vi "LED.vi"(6 "Numbers":dbl[](array[numeric])=[2.0, 4.0, 100.0, 30.0, 2.0, 6.0], 8 "colors":u32[](array[colorbox])=[16712704, 1507583, 65302], 9 "Control_State":T1, 10 "Length":dbl, 11 "Iteration_Num":dbl) -> (3 "Output_Array":u32[](array[numeric]))   [LabVIEW 2020]
uses:
  <vilib>/numeric/Random Number (Range) U64.vi
  af1e4812-ce9e-4321-a641-5b8f74c4ca52.vi
  0c29d166-b99e-4576-9ee3-0d9caf6f3888.vi
  LED_Control_States.ctl
panel:
  in  "Flames":u32[](array[colorbox])=[16711680, 16718848, 16727296, 16733696, 16743168, 16750592, 15706624, 16758784, 16768322, 16776704, 0, 0, 0]
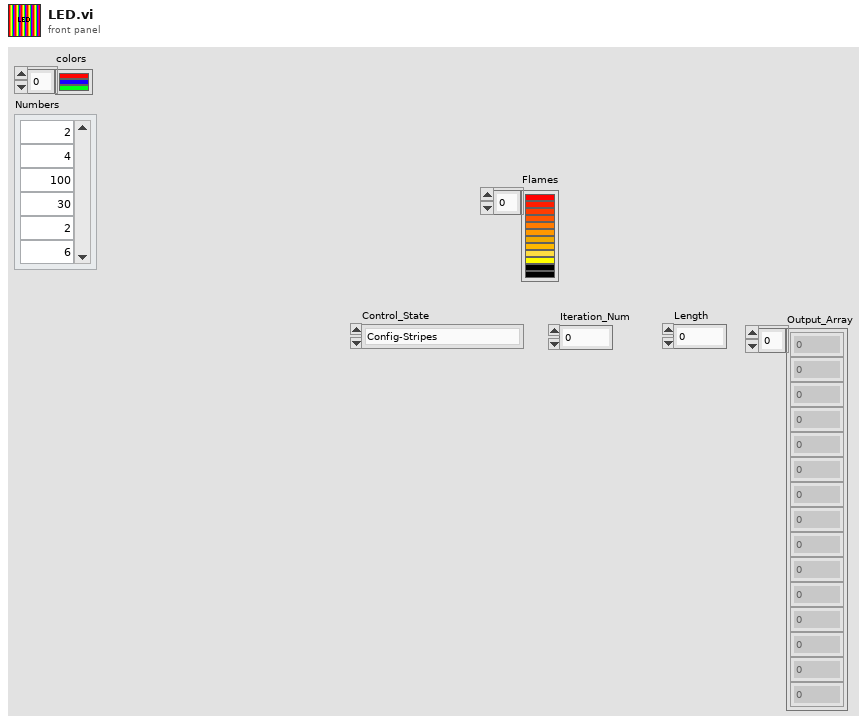
[diagram p1: front panel]
types:
  T1 = typedef "LED_Control_States.ctl" = enum16{"Config-Stripes", "swapperlines", "Rand", "Solid", "Flash-S", "Gradyent", "Move-Stripes", "Org-Rand", "Move-Point-Tail", "Flames", "Fade", "Alt-Colors"}
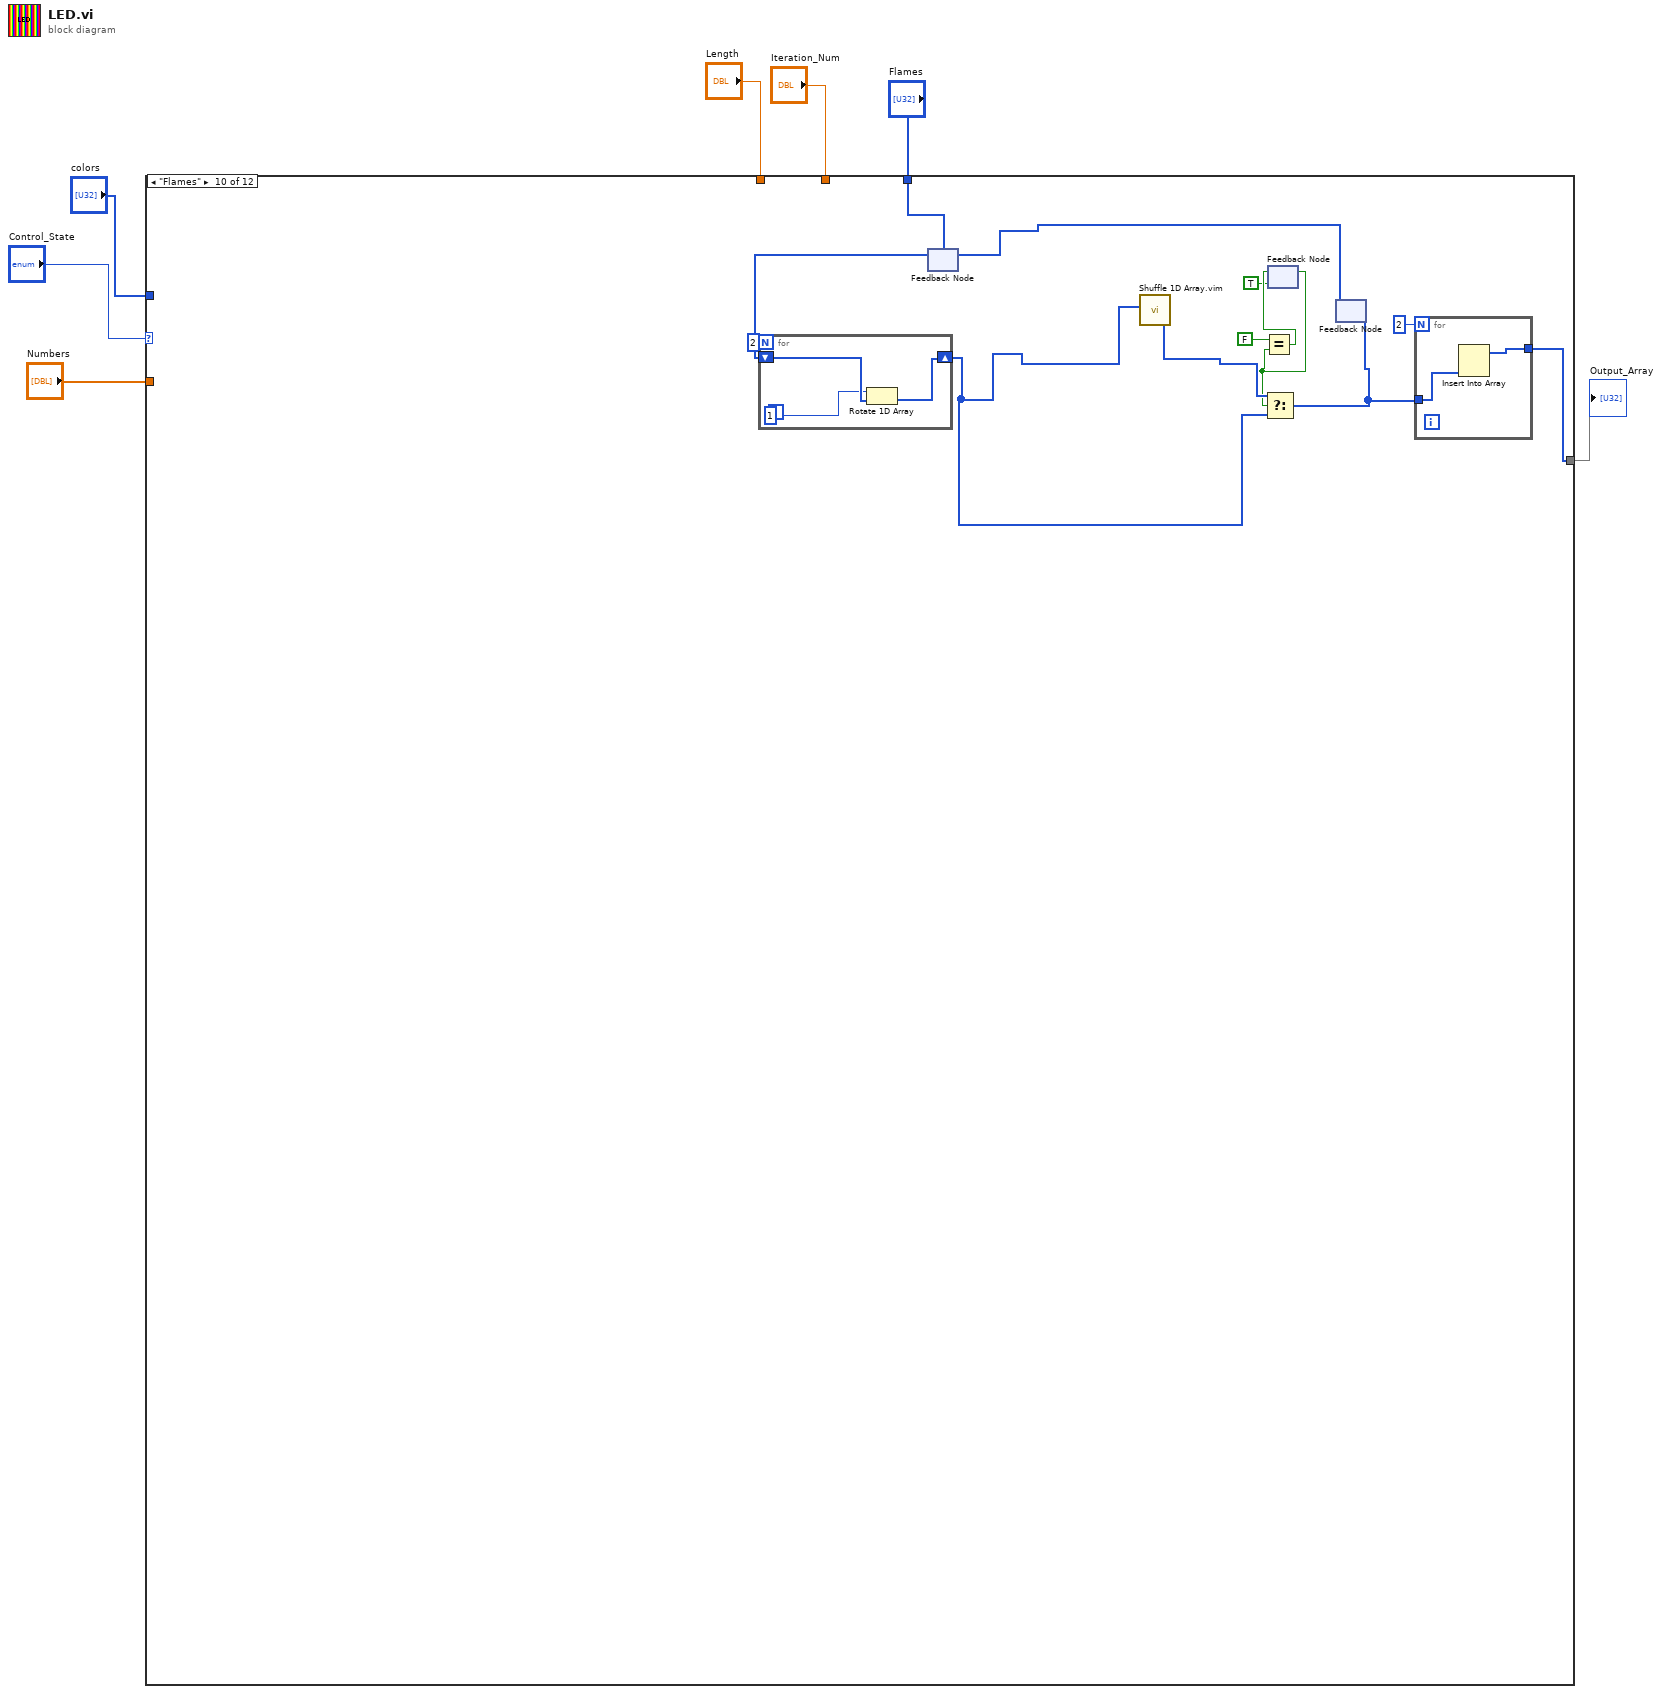
[diagram p0: block diagram]
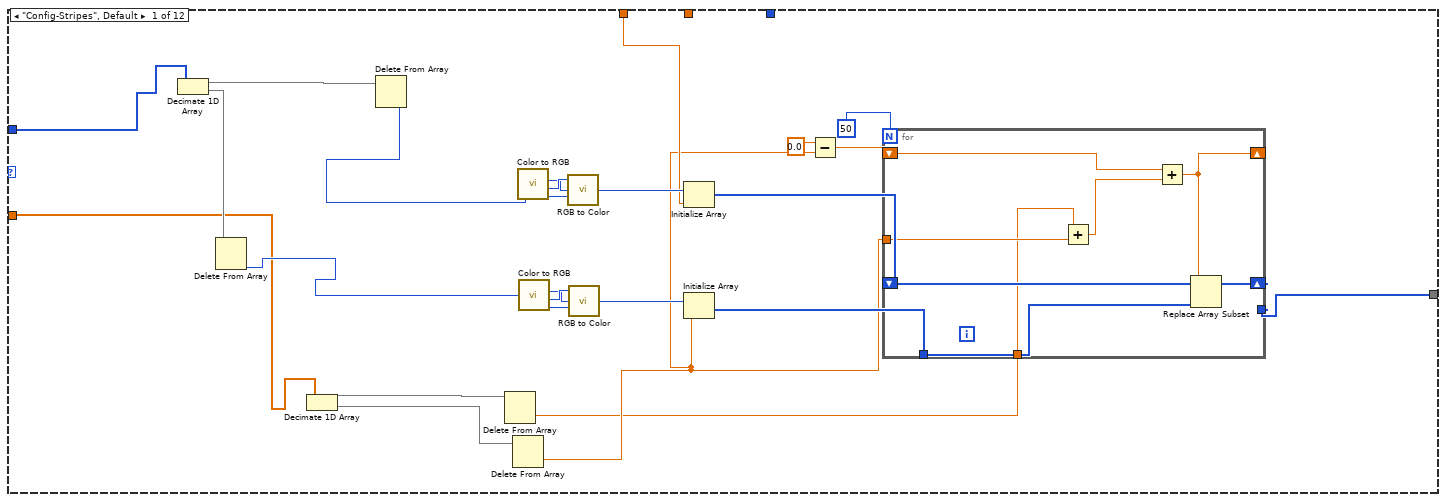
[diagram p2: hidden frame]
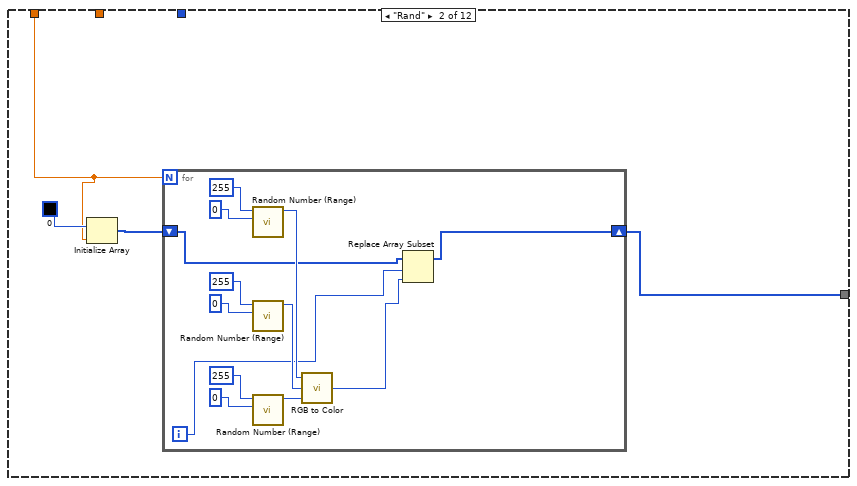
[diagram p3: hidden frame]
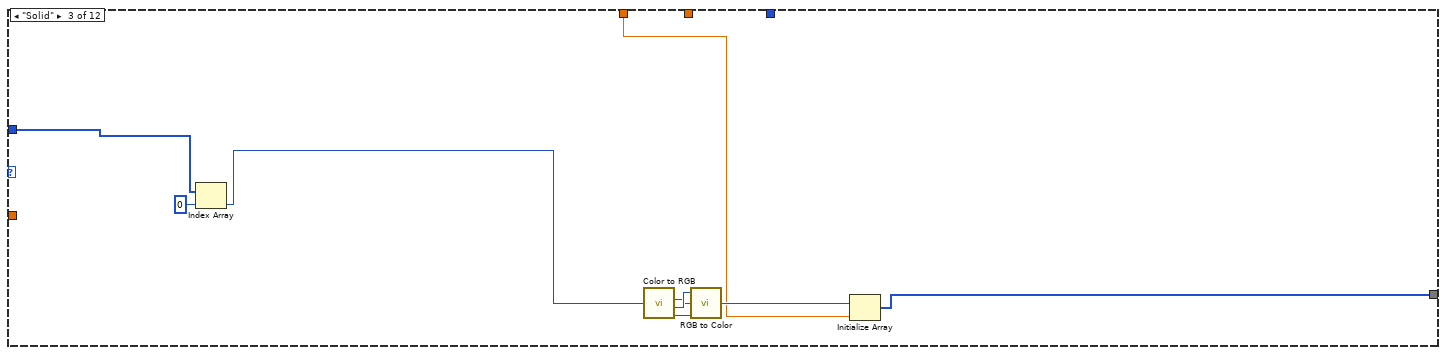
[diagram p4: hidden frame]
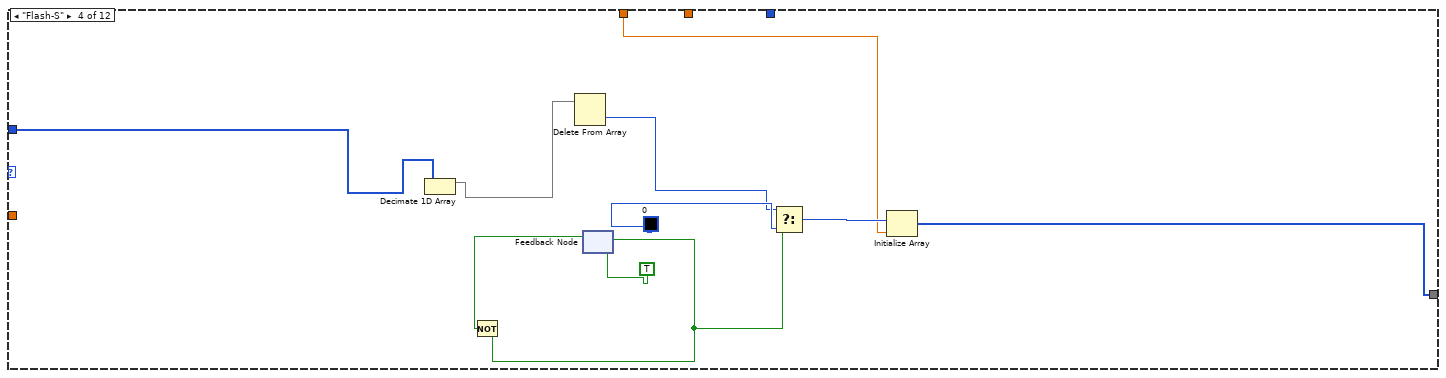
[diagram p5: hidden frame]
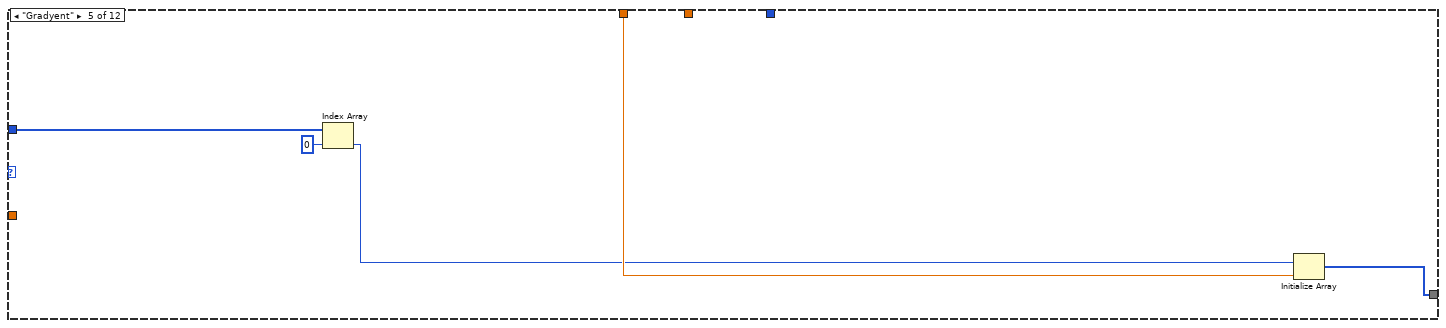
[diagram p6: hidden frame]
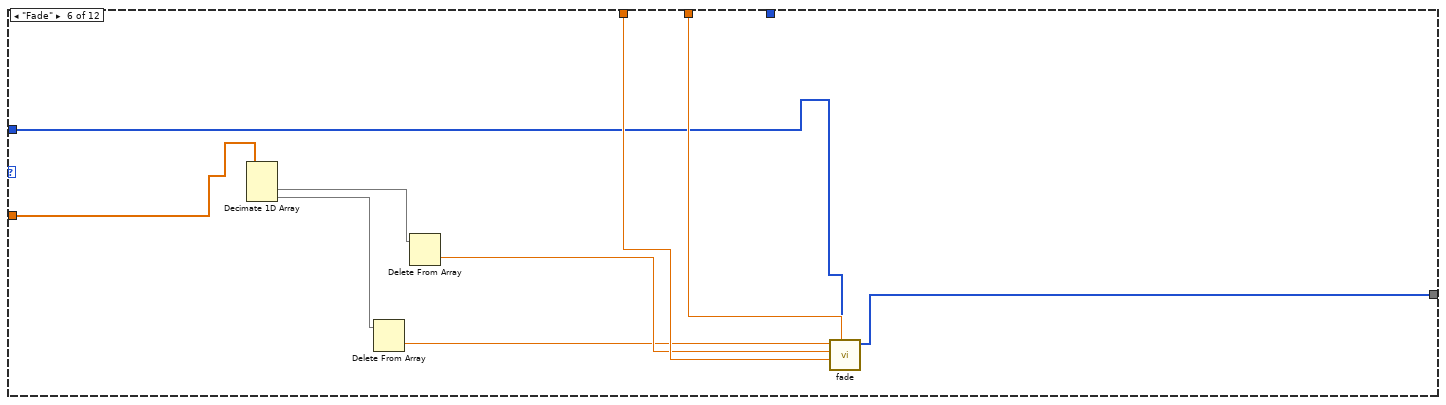
[diagram p7: hidden frame]
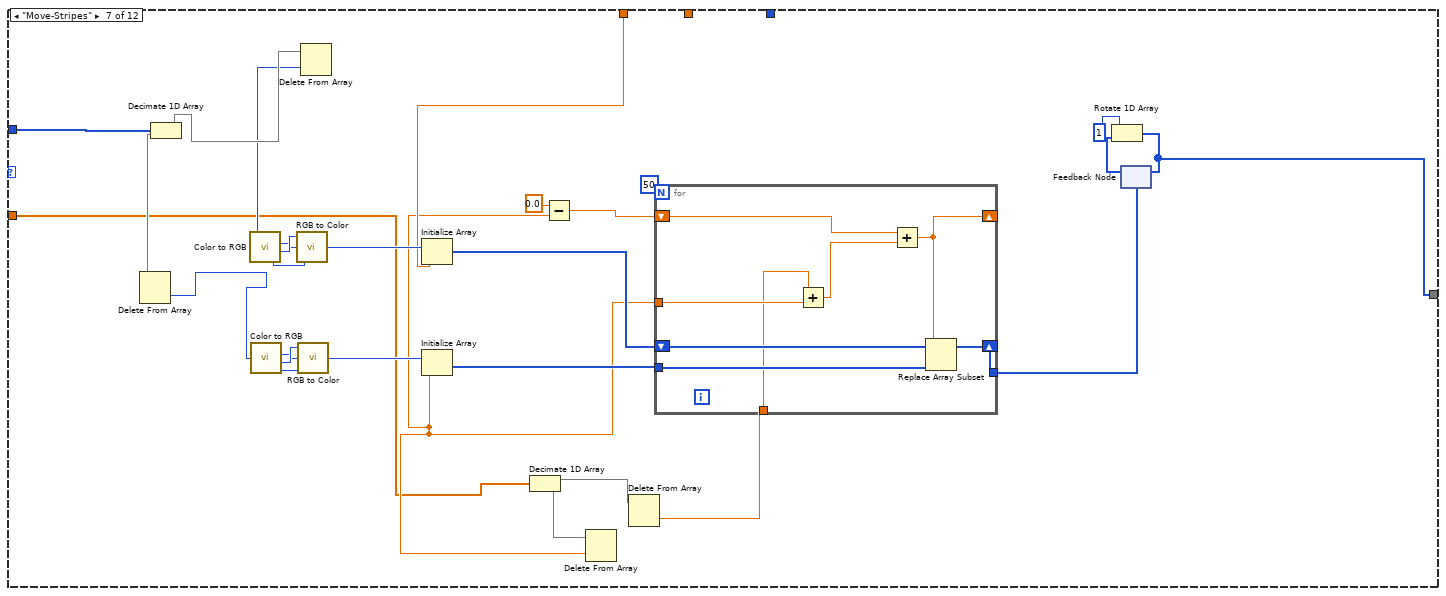
[diagram p8: hidden frame]
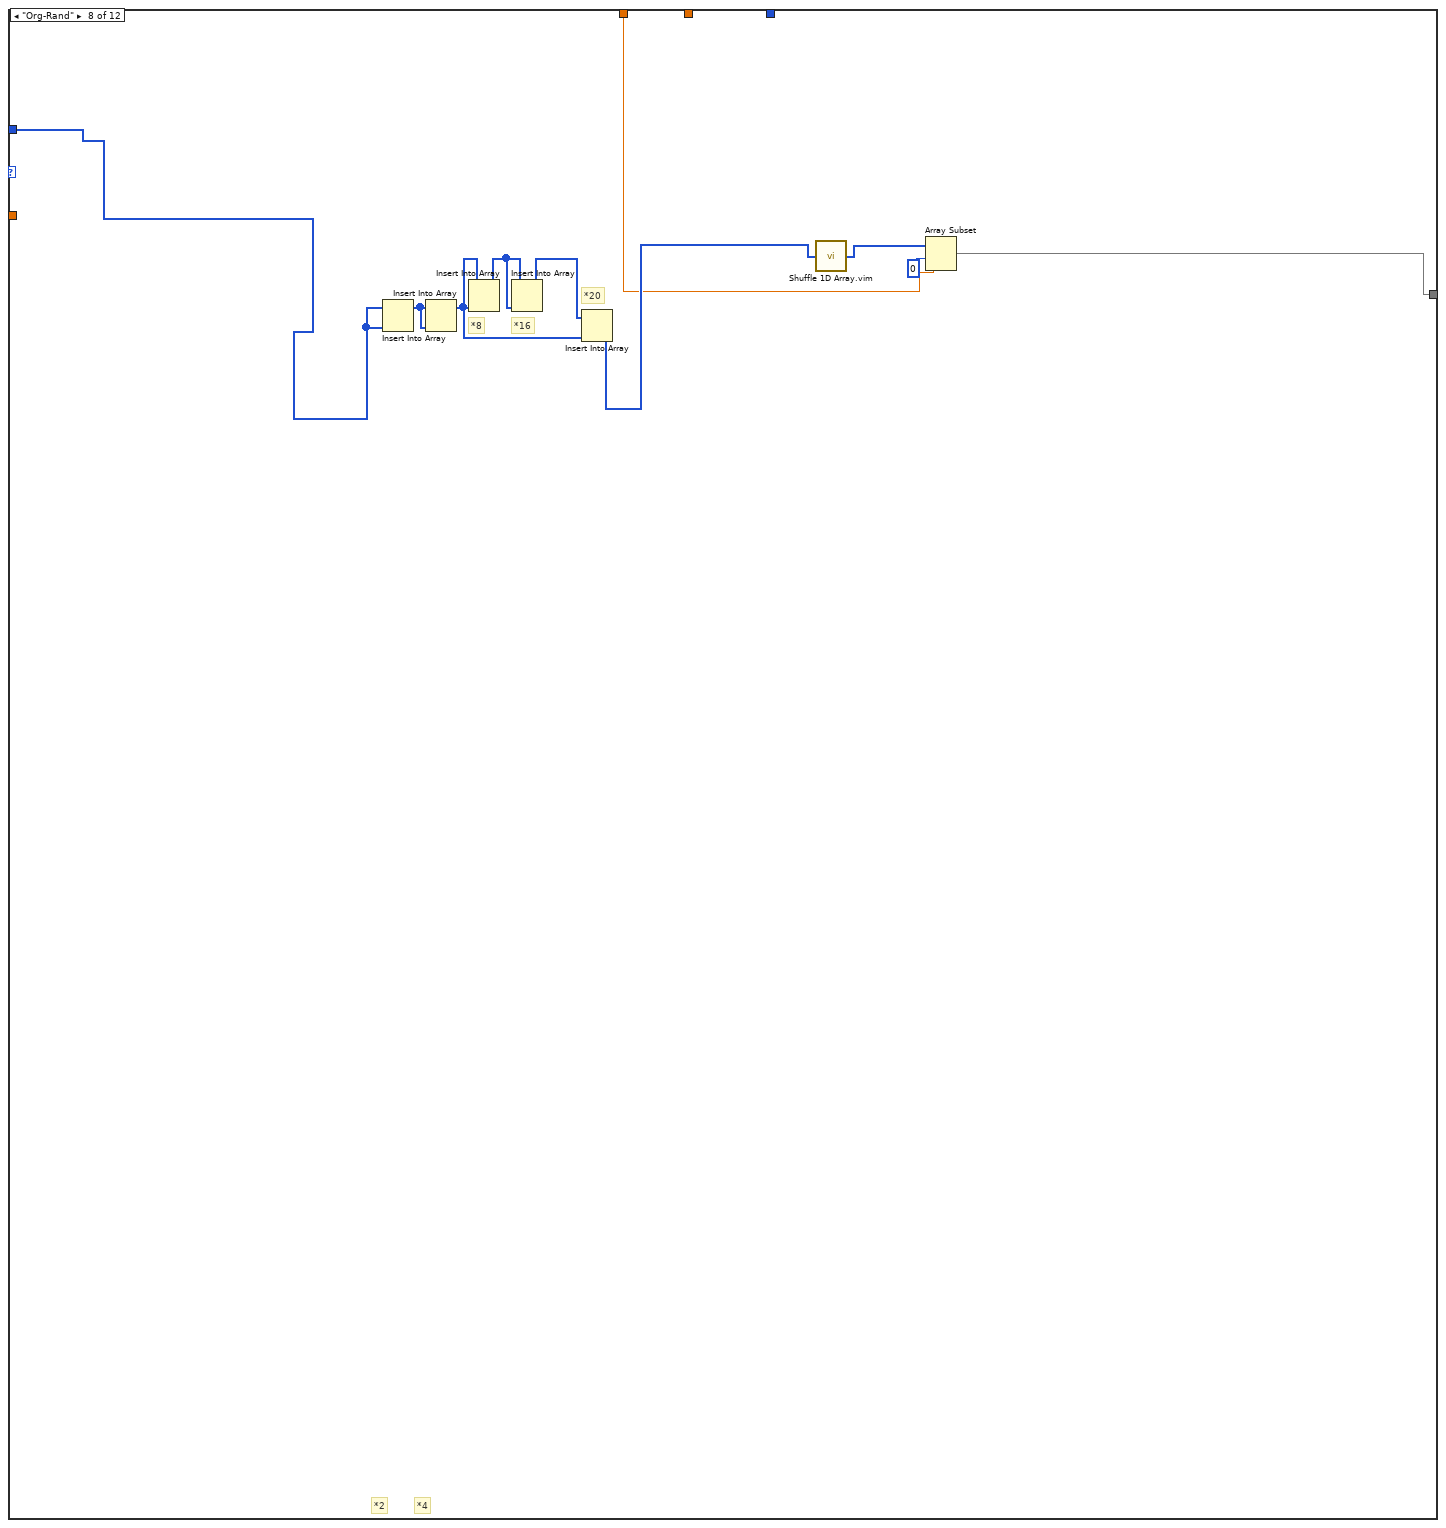
[diagram p9: hidden frame]
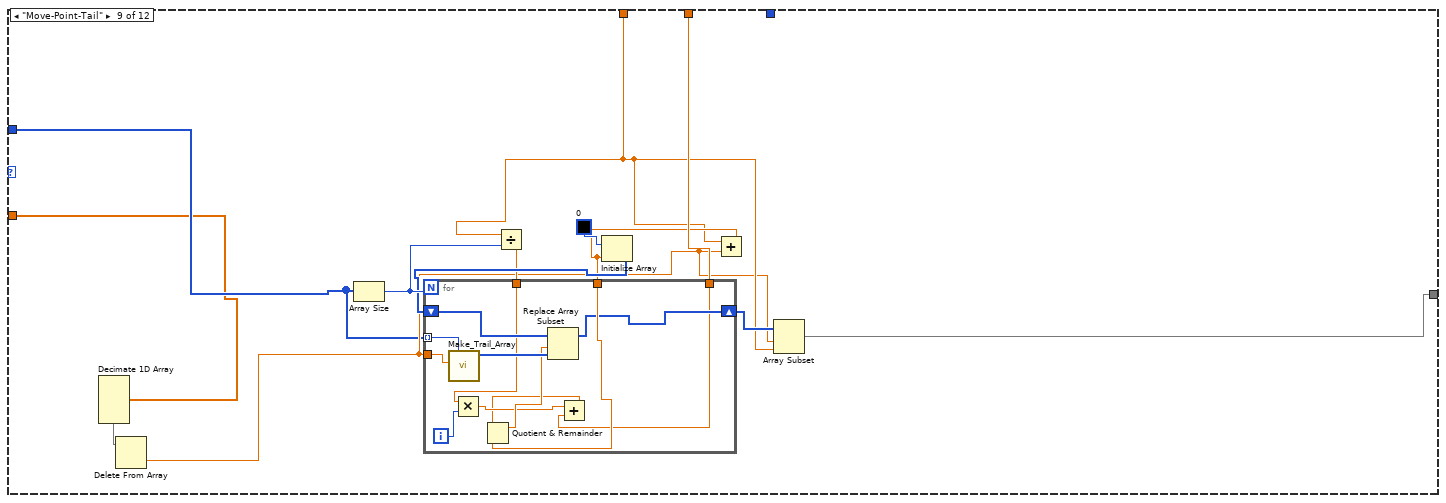
[diagram p10: hidden frame]
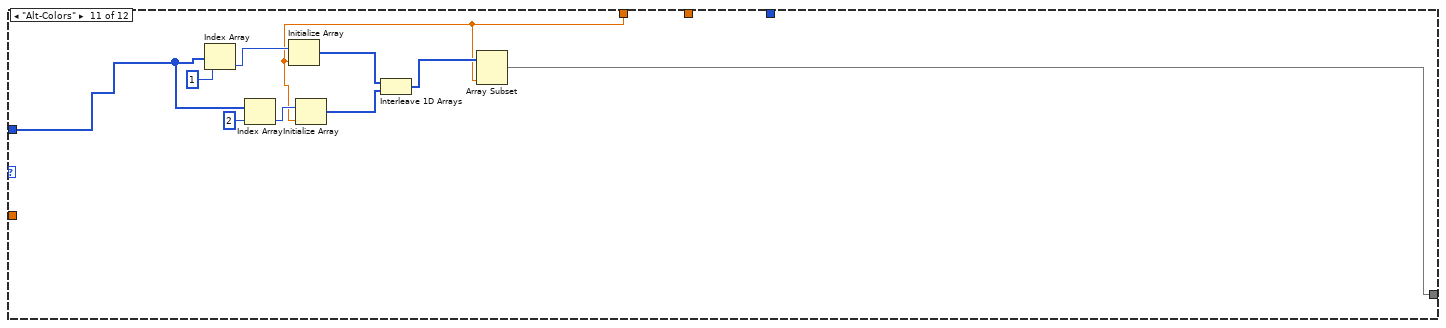
[diagram p11: hidden frame]
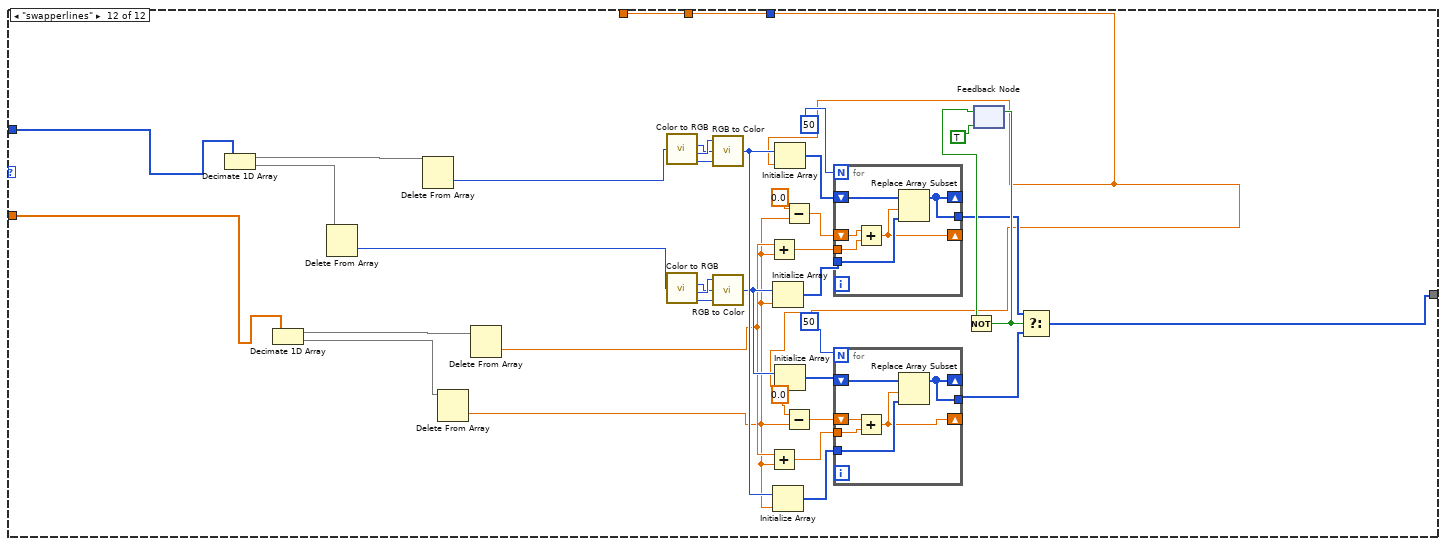
[diagram p12: hidden frame]
diagram:
  n1 = case shown="\"Flames\"" "Control_State" {
    tunnel: [w18 w41 w61 w70 w81 w88 w101 w128 w143 w166 w180 w201] -> w7
    tunnel: "Length" -> [w19 w43 w62 w71 w80 w89 w105 w129 w142 _ w181 w200]
    tunnel: "Iteration_Num" -> [_ _ _ _ _ w90 _ _ w146 _ _ _]
    tunnel: "colors" -> [w9 _ w60 w67 w79 w83 w92 w127 w138 _ w188 w191]
    tunnel: "Numbers" -> [w8 _ _ _ _ w82 w91 _ w137 _ _ w190]
    tunnel: "Flames" -> [_ _ _ _ _ _ _ _ _ w174 _ _]
    frame "Config-Stripes", Default {
      n2 = Decimate 1D Array(w9) -> (w17:u32[], w16:u32[])
      n3 = Delete From Array(array=w16) -> (deleted portion=w15:u32)  [unwired: 2 in, 1 out]
      n4 = Decimate 1D Array(w8) -> (w13:dbl[], w12:dbl[])
      n5 = Delete From Array(array=w17) -> (deleted portion=w14:u32)  [unwired: 2 in, 1 out]
      n6 = Delete From Array(array=w13) -> (deleted portion=w10:dbl)  [unwired: 2 in, 1 out]
      n7 = Delete From Array(array=w12) -> (deleted portion=w11:dbl)  [unwired: 2 in, 1 out]
      n8 = call <vilib>:"Color to RGB.vi"("Color"=w14) -> ("R"=w23:u8, "G"=w24:u8, "B"=w25:u8)  [unwired: 1 out]
      n9 = call <vilib>:"Color to RGB.vi"("Color"=w15) -> ("R"=w26:u8, "G"=w27:u8, "B"=w28:u8)  [unwired: 1 out]
      n10 = call <vilib>:"RGB to Color.vi"("B"=w25, "G"=w23, "R"=w24) -> ("Color"=w22:u32)
      n11 = call <vilib>:"RGB to Color.vi"("B"=w28, "G"=w26, "R"=w27) -> ("Color"=w21:u32)
      n12 = Initialize Array(w22, w19) -> (w31:u32[])
      n13 = Initialize Array(w21, w11) -> (w20:u32[])
      n14 = Subtract(x=0.0, y=w11) -> (x-y=w29:dbl)
      n15 = for {
        N: 50 -> [_]
        shift-right: [w38] -> _
        shift-left: w29 -> [w39]
        tunnel: w20 -> [w40]
        shift-right: [w37] -> _
        shift-left: w31 -> [w36]
        tunnel: [w37] -> w18
        tunnel: w11 -> [w34]
        tunnel: w10 -> [w33]
        n16 = Add(x=w33, y=w34) -> (x+y=w35:dbl)
        n17 = Add(x=w39, y=w35) -> (x+y=w38:dbl)
        n18 = Replace Array Subset(array=w36, new element=w40, index=w38) -> (w37:u32[])
      }
    }
    frame "Rand" {
      n19 = Initialize Array(u32 0, w43) -> (w42:u32[])
      n20 = for {
        N: w43 -> [_]
        shift-right: [w45] -> w41
        shift-left: w42 -> [w46]
        i -> [w48]
        n21 = call-poly <vilib>:"Random Number (Range).vi"("lower bound (0)"=u64 0, "upper bound (100)"=u64 255) -> ("number"=w57:u64)  [unwired: 9 in]
        n22 = call-poly <vilib>:"Random Number (Range).vi"("lower bound (0)"=u64 0, "upper bound (100)"=u64 255) -> ("number"=w56:u64)  [unwired: 9 in]
        n23 = call-poly <vilib>:"Random Number (Range).vi"("lower bound (0)"=u64 0, "upper bound (100)"=u64 255) -> ("number"=w55:u64)  [unwired: 9 in]
        n24 = call <vilib>:"RGB to Color.vi"("B"=w55, "G"=w56, "R"=w57) -> ("Color"=w47:u32)
        n25 = Replace Array Subset(array=w46, new element=w47, index=w48) -> (w45:u32[])
      }
    }
    frame "Solid" {
      n26 = Index Array(array=w60, index=0) -> (element=w59:u32)
      n27 = call <vilib>:"Color to RGB.vi"("Color"=w59) -> ("R"=w64:u8, "G"=w65:u8, "B"=w66:u8)  [unwired: 1 out]
      n28 = call <vilib>:"RGB to Color.vi"("B"=w66, "G"=w64, "R"=w65) -> ("Color"=w63:u32)
      n29 = Initialize Array(w63, w62) -> (w61:u32[])
    }
    frame "Flash-S" {
      n30 = Decimate 1D Array(w67) -> (w69:u32[])  [unwired: 1 out]
      n31 = Delete From Array(array=w69) -> (deleted portion=w68:u32)  [unwired: 2 in, 1 out]
      n32 = feedback #1(TRUE) -> (w74:bool)
      n33 = Not(x=w74) -> (.not. x?=w73:bool)
      n34 = feedback-in #1(w73) -> ()
      n35 = Select(t=w68, s=w73, f=u32 0) -> (s? t:f=w76:u32)
      n36 = Initialize Array(w76, w71) -> (w70:u32[])
    }
    frame "Gradyent" {
      n37 = Index Array(array=w79, index=0) -> (element=w77:u32)
      n38 = Initialize Array(w77, w80) -> (w81:u32[])
    }
    frame "Fade" {
      n39 = Decimate 1D Array(w82) -> (w87:dbl[], w85:dbl[])  [unwired: 3 out]
      n40 = Delete From Array(array=w85) -> (deleted portion=w84:dbl)  [unwired: 2 in, 1 out]
      n41 = Delete From Array(array=w87) -> (deleted portion=w86:dbl)  [unwired: 2 in, 1 out]
      n42 = call "fade.vi"("Iteration_Num"=w90, "Color Array"=w83, "Length"=w89, "fade constant"=w86, "Wait_Constant"=w84) -> ("Output_Array"=w88:u32[])  [unwired: 6 in]
    }
    frame "Move-Stripes" {
      n43 = Decimate 1D Array(w92) -> (w100:u32[], w97:u32[])
      n44 = Delete From Array(array=w97) -> (deleted portion=w98:u32)  [unwired: 2 in, 1 out]
      n45 = call <vilib>:"Color to RGB.vi"("Color"=w98) -> ("R"=w112:u8, "G"=w113:u8, "B"=w114:u8)  [unwired: 1 out]
      n46 = call <vilib>:"RGB to Color.vi"("B"=w114, "G"=w112, "R"=w113) -> ("Color"=w107:u32)
      n47 = Delete From Array(array=w100) -> (deleted portion=w99:u32)  [unwired: 2 in, 1 out]
      n48 = call <vilib>:"Color to RGB.vi"("Color"=w99) -> ("R"=w109:u8, "G"=w110:u8, "B"=w111:u8)  [unwired: 1 out]
      n49 = call <vilib>:"RGB to Color.vi"("B"=w111, "G"=w109, "R"=w110) -> ("Color"=w108:u32)
      n50 = Initialize Array(w108, w105) -> (w117:u32[])
      n51 = Decimate 1D Array(w91) -> (w96:dbl[], w95:dbl[])
      n52 = Delete From Array(array=w95) -> (deleted portion=w94:dbl)  [unwired: 2 in, 1 out]
      n53 = Initialize Array(w107, w94) -> (w106:u32[])
      n54 = Subtract(x=0.0, y=w94) -> (x-y=w115:dbl)
      n55 = Delete From Array(array=w96) -> (deleted portion=w93:dbl)  [unwired: 2 in, 1 out]
      n56 = for {
        N: 50 -> [_]
        shift-right: [w124] -> _
        shift-left: w115 -> [w125]
        tunnel: w106 -> [w126]
        shift-right: [w123] -> _
        shift-left: w117 -> [w122]
        tunnel: [w123] -> w104
        tunnel: w94 -> [w120]
        tunnel: w93 -> [w119]
        n57 = Add(x=w119, y=w120) -> (x+y=w121:dbl)
        n58 = Add(x=w125, y=w121) -> (x+y=w124:dbl)
        n59 = Replace Array Subset(array=w122, new element=w126, index=w124) -> (w123:u32[])
      }
      n60 = feedback #2(w104) -> (w102:u32[])
      n61 = Rotate 1D Array(1:w102, 2:1 ("n")) -> (0:w101:u32[])
      n62 = feedback-in #2(w101) -> ()
    }
    frame "Org-Rand" {
      # "*20"
      # "*16"
      # "*8"
      # "*4"
      # "*2"
      n63 = Insert Into Array(array=w127, new element=w127) -> (w136:u32[])  [unwired: 1 in]
      n64 = Insert Into Array(array=w136, new element=w136) -> (w134:u32[])  [unwired: 1 in]
      n65 = Insert Into Array(array=w134, new element=w134) -> (w135:u32[])  [unwired: 1 in]
      n66 = Insert Into Array(array=w135, new element=w135) -> (w133:u32[])  [unwired: 1 in]
      n67 = Insert Into Array(array=w133, new element=w134) -> (w132:u32[])  [unwired: 1 in]
      n68 = call "Shuffle 1D Array.vim"("array"=w132) -> ("shuffled array"=w131:u32[])  [unwired: 4 in]
      n69 = Array Subset(array=w131, index=0, length=w129) -> (w128:u32[])
    }
    frame "Move-Point-Tail" {
      n70 = Decimate 1D Array(w137) -> (w140:dbl[])  [unwired: 5 out]
      n71 = Delete From Array(array=w140) -> (deleted portion=w139:dbl)  [unwired: 2 in, 1 out]
      n72 = Array Size(array=w138) -> (size(s)=w149:i32)
      n73 = Divide(x=w142, y=w149) -> (x/y=w141:dbl)
      n74 = Add(x=w142, y=w139) -> (x+y=w145:dbl)
      n75 = Initialize Array(u32 0, w145) -> (w147:u32[])
      n76 = for {
        N: w149 -> [_]
        tunnel: w138 -> [w161] mode=indexing
        shift-right: [w156] -> w144
        shift-left: w147 -> [w160]
        tunnel: w146 -> [w151]
        tunnel: w145 -> [w157]
        tunnel: w139 -> [w155]
        tunnel: w141 -> [w153]
        i -> [w154]
        n77 = call "Make_Trail_Array.vi"("Trail_Length"=w155, "Dot_Color"=w161) -> ("Trail_Array"=w159:u32[])  [unwired: 9 in]
        n78 = Multiply(x=w153, y=w154) -> (x*y=w152:dbl)
        n79 = Add(x=w152, y=w151) -> (x+y=w150:dbl)
        n80 = Quotient & Remainder(x=w150, y=w157) -> (x-y*floor(x/y)=w158:dbl)  [unwired: 1 out]
        n81 = Replace Array Subset(array=w160, new element=w159, index=w158) -> (w156:u32[])
      }
      n82 = Array Subset(array=w144, index=w139, length=w142) -> (w143:u32[])
    }
    frame "Flames" {
      n83 = feedback #3(w174) -> (w163:u32[])
      n84 = for {
        N: 2 -> [_]
        shift-right: [w175] -> w172
        shift-left: w163 -> [w177]
        n85 = Rotate 1D Array(1:w177, 2:1 ("n")) -> (0:w175:u32[])
      }
      n86 = call "Shuffle 1D Array.vim"("array"=w172) -> ("shuffled array"=w173:u32[])  [unwired: 4 in]
      n87 = feedback #4(TRUE) -> (w169:bool)
      n88 = Equal?(x=FALSE, y=w169) -> (x = y?=w170:bool)
      n89 = Select(t=w173, s=w169, f=w172) -> (s? t:f=w165:u32[])
      n90 = feedback-in #4(w170) -> ()
      n91 = feedback-in #5(w165) -> ()
      n92 = feedback #5() -> (w171:u32[])  [unwired: 1 in]
      n93 = feedback-in #3(w171) -> ()
      n94 = for {
        N: 2 -> [_]
        tunnel: [w179] -> w166
        tunnel: w165 -> [w178]
        n95 = Insert Into Array(array=w178, new element=w178) -> (w179:u32[])  [unwired: 1 in]
      }
    }
    frame "Alt-Colors" {
      n96 = Index Array(array=w188, index=1) -> (element=w186:u32)
      n97 = Index Array(array=w188, index=2) -> (element=w185:u32)
      n98 = Initialize Array(w186, w181) -> (w184:u32[])
      n99 = Initialize Array(w185, w181) -> (w183:u32[])
      n100 = Interleave 1D Arrays(w184, w183) -> (w182:u32[])
      n101 = Array Subset(array=w182, length=w181) -> (w180:u32[])  [unwired: 1 in]
    }
    frame "swapperlines" {
      n102 = Decimate 1D Array(w191) -> (w199:u32[], w197:u32[])
      n103 = Decimate 1D Array(w190) -> (w195:dbl[], w194:dbl[])
      n104 = Delete From Array(array=w197) -> (deleted portion=w196:u32)  [unwired: 2 in, 1 out]
      n105 = Delete From Array(array=w199) -> (deleted portion=w198:u32)  [unwired: 2 in, 1 out]
      n106 = Delete From Array(array=w194) -> (deleted portion=w192:dbl)  [unwired: 2 in, 1 out]
      n107 = Delete From Array(array=w195) -> (deleted portion=w193:dbl)  [unwired: 2 in, 1 out]
      n108 = call <vilib>:"Color to RGB.vi"("Color"=w198) -> ("R"=w207:u8, "G"=w208:u8, "B"=w209:u8)  [unwired: 1 out]
      n109 = call <vilib>:"Color to RGB.vi"("Color"=w196) -> ("R"=w203:u8, "G"=w204:u8, "B"=w205:u8)  [unwired: 1 out]
      n110 = call <vilib>:"RGB to Color.vi"("B"=w209, "G"=w207, "R"=w208) -> ("Color"=w206:u32)
      n111 = call <vilib>:"RGB to Color.vi"("B"=w205, "G"=w203, "R"=w204) -> ("Color"=w202:u32)
      n112 = Add(x=w193, y=w192) -> (x+y=w221:dbl)
      n113 = Add(x=w193, y=w192) -> (x+y=w211:dbl)
      n114 = Initialize Array(w202, w192) -> (w225:u32[])
      n115 = Initialize Array(w206, w192) -> (w215:u32[])
      n116 = Initialize Array(w206, w200) -> (w224:u32[])
      n117 = Initialize Array(w202, w200) -> (w214:u32[])
      n118 = Subtract(x=0.0, y=w192) -> (x-y=w222:dbl)
      n119 = Subtract(x=0.0, y=w192) -> (x-y=w212:dbl)
      n120 = for {
        N: 50 -> [_]
        shift-right: [w236] -> _
        shift-left: w222 -> [w237]
        tunnel: w225 -> [w238]
        shift-right: [w235] -> _
        shift-left: w224 -> [w234]
        tunnel: [w235] -> w217
        tunnel: w221 -> [w233]
        n121 = Add(x=w237, y=w233) -> (x+y=w236:dbl)
        n122 = Replace Array Subset(array=w234, new element=w238, index=w236) -> (w235:u32[])
      }
      n123 = for {
        N: 50 -> [_]
        shift-right: [w230] -> _
        shift-left: w212 -> [w231]
        tunnel: w215 -> [w232]
        shift-right: [w229] -> _
        shift-left: w214 -> [w228]
        tunnel: [w229] -> w210
        tunnel: w211 -> [w227]
        n124 = Add(x=w231, y=w227) -> (x+y=w230:dbl)
        n125 = Replace Array Subset(array=w228, new element=w232, index=w230) -> (w229:u32[])
      }
      n126 = feedback #6(TRUE) -> (w219:bool)
      n127 = Not(x=w219) -> (.not. x?=w218:bool)
      n128 = feedback-in #6(w218) -> ()
      n129 = Select(t=w217, s=w218, f=w210) -> (s? t:f=w201:u32[])
    }
  }
  "Output_Array" <- w7
